vi "run.vi"() -> ()   [LabVIEW 2017]
uses:
  <vilib>/Analysis/Matrix/Datatypes/RealMatrix.ctl
  <vilib>/Simulation/Scripting/Companion Diagram/SimConfigNode/SimParams.ctl
  <vilib>/Simulation/Scripting/Companion Diagram/SimConfigNode/_simSolvers.ctl
  <vilib>/Simulation/Implementation/Shared/SIMSCR Execution Mode.ctl
  <vilib>/Simulation/Param Hierarchy/Typedefs/SIMPH Param Control Actions.ctl
  <vilib>/Simulation/Implementation/Shared/NILVSim_ParamChanged.vi
  <vilib>/Simulation/Implementation/Shared/NILVSIM_BeginStep.vi
  <vilib>/Simulation/SignalDisplay/Implementation/NILVSim Time Waveform.llb/SIM Time Waveform (vector).vi
  <vilib>/Simulation/SignalDisplay/Implementation/NILVSim Time Waveform.llb/SIM Time Waveform (scalar).vi
  <vilib>/Simulation/Implementation/Shared/SIM Is Init or Final Stage.vi
  <vilib>/Simulation/Implementation/Shared/NILVSim_Manager.vi
  <vilib>/Utility/error.llb/Clear Errors.vi
  <vilib>/Simulation/Implementation/Shared/NILVSim_FinalizeModel.vi
  <vilib>/picture/3D Picture Control/Object/Create Object (name).vi
  <vilib>/Analysis/7linalg.llb/Create Special Real Matrix.vi
  <vilib>/addons/Control Design/_Stochastic Systems/Stochastic Systems.llb/CD Construct Stochastic Model (Numeric).vi
  <vilib>/Simulation/Implementation/Shared/SIM Unbundle Sim Info.vi
  <vilib>/Simulation/Implementation/Shared/NILVSim_Initialize.vi
  SubVI/disturbance.vi
  <vilib>/addons/Control Design/_Stochastic Systems/Stochastic Systems.llb/CD Construct Noise Model.vi
  <vilib>/addons/Control Design/_Stochastic Systems/Stochastic Systems.llb/CD Construct Noise Model (Numeric).vi
  <vilib>/addons/Control Design/_State Feedback Control/State Feedback Control.llb/CD Linear Quadratic Regulator.vi
  <vilib>/addons/Control Design/_State Feedback Control/State Feedback Control.llb/State Feedback Control SubVis/cd_Linear Quadratic Regulator.vi
  <vilib>/addons/Control Design/_Implementation/CD State Feedback Controller.vi
  <vilib>/addons/Control Design/_Implementation/CD State Feedback Controller (Multiple Outputs).vi
  <vilib>/Simulation/Utility/Implementation/NILVSim Get Time and IsAcceptedStep.vi
  <vilib>/Simulation/DiscreteLinear/Implementation/NILVSim Discrete Stochastic State Space.llb/SIM Discrete Stochastic State Space External Indirect Distributor Sim.vi
  SubVI/lib/instrument.vi
  SubVI/3DMotion.vi
  <vilib>/Simulation/Estimation/Implementation/NILVSim Discrete Kalman Filter.llb/SIM Disc KF Pred and Corr with Pred Gain with Checking Indirect Distributor Sim.vi
  <vilib>/Simulation/DiscreteLinear/Implementation/NILVSim Discrete Stochastic State Space.llb/SIM Discrete Stochastic State Space External Indirect Collector Sim.vi
  <vilib>/Simulation/Estimation/Implementation/NILVSim Discrete Kalman Filter.llb/SIM Disc KF Pred and Corr with Pred Gain with Checking Indirect Collector Sim.vi
  <vilib>/Simulation/Implementation/Shared/SIMSH Read Queue.vi
  <vilib>/Simulation/Implementation/Shared/NILVSim_GetModelError.vi
  <vilib>/Simulation/Implementation/Shared/SIM Bundle Sim Info.vi
  <vilib>/Simulation/Scripting/Companion Diagram/SimConfigNode/SimDog.xnode
  <vilib>/Simulation/Implementation/XNodeFramework/SimXNode/SimX.xnode
  <vilib>/picture/3D Picture Control/NI_3D Picture Control.lvlib
  <vilib>/addons/Control Design/_State Feedback Control/NI_CD_State Feedback Control.lvlib
  <vilib>/addons/Control Design/_Stochastic Systems/NI_CD_Stochastic Systems.lvlib
  <vilib>/Analysis/NI_AALPro.lvlib
  <vilib>/addons/Control Design/_Utility/NI_CD_Model Viewer.lvlib
  <vilib>/addons/Control Design/_Implementation/NI_CD_Implementation.lvlib
  <vilib>/Simulation/Estimation/Implementation/NILVSim Discrete Kalman Filter.llb/SIM Disc KF Pred and Corr with Pred Gain with Checking Indirect Sim.vi
  <vilib>/Simulation/DiscreteLinear/Implementation/NILVSim Discrete Stochastic State Space.llb/NILVSim Discrete Stochastic State Space External Indirect Sim.vi
  <vilib>/Simulation/Implementation/Shared/NI_SIM_Implementation.lvlib
  <vilib>/Analysis/Matrix/NI_Matrix.lvlib
panel:
  in  "Optimal States (x1, x2, x3, x4, x5, x6)":dbl[](array[knob])=[1.0, 1.0, 1.0, 1.0, 1.0, 1.0] scale=0.01..100.0
  in  "Optimal Energy (u1, u2, u3)":dbl[](array[knob])=[1.0, 1.0, 1.0] scale=0.01..100.0
  out "State x(k+1)":dbl[](array[numeric])
  in  "Jz":dbl=0.0071
  in  "Jy":dbl=0.0038
  in  "Jx":dbl=0.0038
  in  "kr":dbl=0.00064
  in  "Pitch":dbl[](array[slide])=[0.0] scale=-30.0..60.0
  in  "Roll":dbl[](array[slide])=[0.0] scale=-89.0..89.0
  in  "Yaw S.P.":dbl[](array[slide])=[0.0] scale=-179.0..179.0
  in  "Orientation-Rate":dbl[](array[slide])=[0.0, 0.0, 0.0] scale=0.0..10.0
  out "Control Signals":waveform(dbl)[](graph)
  out "output cluster":T1 {"rotate"."pitch" scale=-30.0..60.0; "rotate"."roll" scale=-89.0..89.0; "rotate"."yaw" scale=-179.0..179.0}
  out "Yaw Error":waveform(dbl)[](graph)
  out "Pitch Error":waveform(dbl)(graph)={"t0"=timestamp(9343.2 s since 1904-01-01), "dt"=1.0, "Y"=[0.2633720690985406]}
  out "Roll Error":waveform(dbl)(graph)={"t0"=timestamp(9343.2 s since 1904-01-01), "dt"=1.0, "Y"=[0.2633720690985406]}
  out "Process Noise w(k)":dbl[](array[numeric])
  in  "Tab Control":enum32{"Model", "LQG"}(tab)
  out "Equation":picture
  out "Controller Action":dbl[](array[numeric]) format="%#.2g"
  out "Rv":T2
  in  "Convariance V":dbl(slide)=0.96 scale=0.0..1.0
  in  "Convariance W":dbl(slide)=0.96 scale=0.0..1.0
  out "Qw":T2
  in  "E{v}":dbl[](array[knob])=[0.96, 0.96, 0.96] scale=0.0..1.0
  in  "E{w}":dbl[](array[knob])=[0.96, 0.96, 0.96] scale=0.0..1.0
  in  "Initialize":bool
  out "Output y(t)":dbl[](array[numeric])
  out "Estimate xhat(k|k)":dbl[](array[numeric])
  out "Action u(k)":dbl[](array[numeric]) format="%#.2g"
  in  "Boolean 3":bool
  out "D(k)":dbl[](array[numeric])
  out "Setpoints_":dbl[](array[numeric])
  out "Yaw S.P. 2":dbl
  out "Waveform Yaw":waveform(dbl)[](graph)
  out "Waveform Pitch":waveform(dbl)[](graph)
  out "Pitch S.P.":dbl
  out "Roll S.P.":dbl
  out "Roll P.V.":dbl
  out "Waveform Roll":waveform(dbl)[](graph)
  in  "Switch\nController":bool
  out "pict out":picture
  out "Yaw P.V.":dbl
  out "Pitch P.V.":dbl
  out "3D Picture Control":refnum<vi>(3d-picture)
  # "References- Setpoints: Orientations, Angular Rates"
  # "N-Roll"
  # "N-Pitch"
  # "N-Yaw"
  # "Roll\nPitch\nYaw"
  # "Setpoints"
  # "u2\nu3 \nu4"
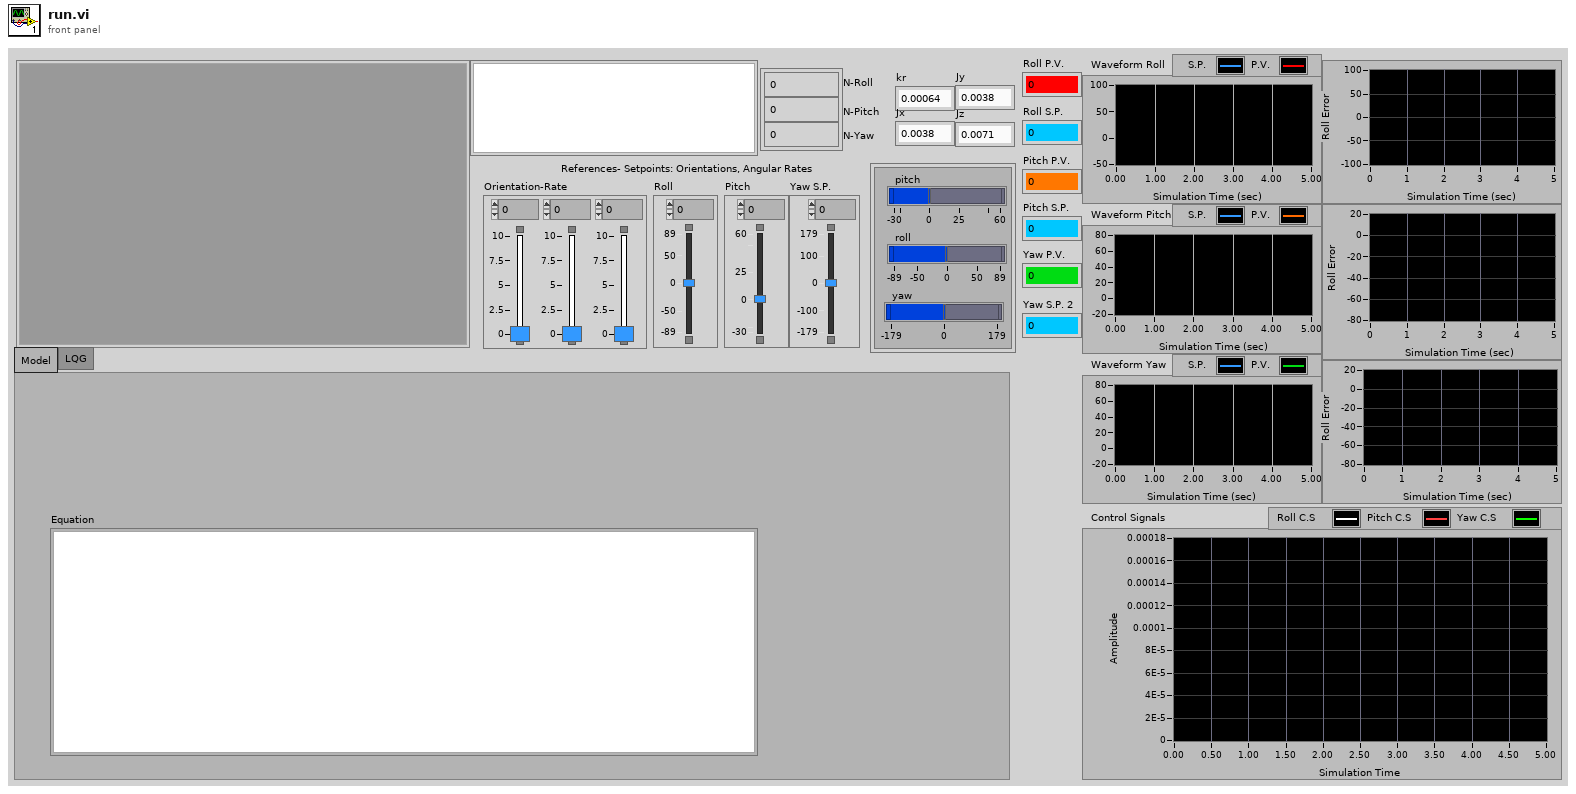
[diagram p1: front panel]
types:
  T1 = cluster{"control stick":cluster{"roll":i32, "pitch":i32}, "rotate":cluster{"pitch":dbl, "roll":dbl, "yaw":dbl}, "pos":cluster{"x":dbl, "y":dbl, "z":i32}}
  T2 = typedef "NI_Matrix.lvlib/RealMatrix.ctl" = dbl[][]
  T3 = typedef "NI_CD_Stochastic Systems.lvlib/cd_Stochastic State-Space Model.ctl" = cluster{"Sampling Time (s)":dbl, "G":dbl[][], "B":dbl[][], "A":dbl[][], "C":dbl[][], "D":dbl[][], "H":dbl[][]}
  T4 = typedef "NI_LinSys_Model Typedefs.lvlib/CD State Space Model (MIMO).ctl" = cluster{"properties":T5, "A":dbl[][], "B":dbl[][], "C":dbl[][], "D":dbl[][], "StateNames":string[], "Transport Delay":dbl[][]}
  T5 = typedef "NI_LinSys_Model Typedefs.lvlib/CD General Elements.ctl" = cluster{"Model name":string, "Input names":string[], "Output names":string[], "Input Delays":dbl[], "Output Delays":dbl[], "Sampling Time":dbl, "Notes":string}
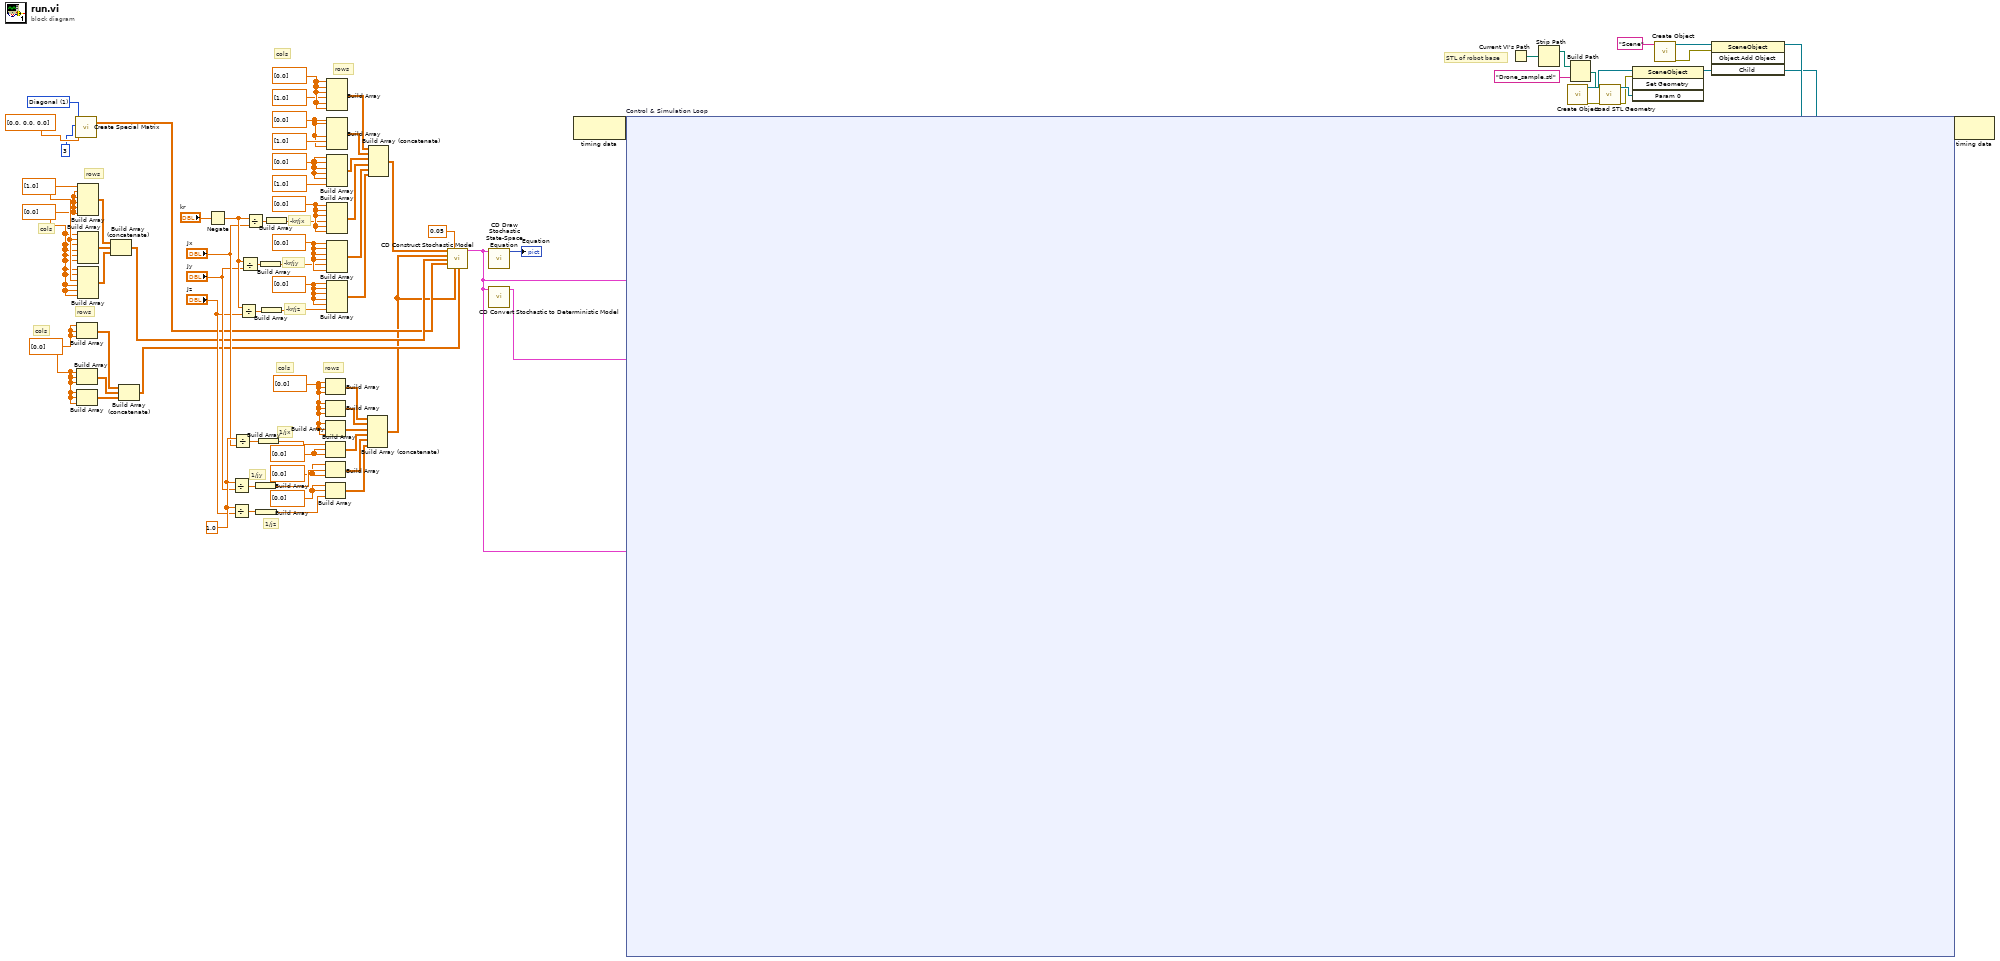
[diagram p0: block diagram]
diagram:
  w14 = dbl[] [0.0] ("element")
  w19 = dbl[] [1.0] ("element")
  w18 = dbl[] [0.0] ("element")
  w26 = 1 items=["Identity", "Diagonal", "Toepliz", "Vandermonde", "Companion", "Hankel", "Hadamard", "Wilkinson", "Hilbert", "Inverse Hilbert", "Rosser", "Pascal"] ("matrix type")
  w30 = 1.0 ("x")
  w34 = dbl[] [0.0] ("element")
  w35 = dbl[] [0.0] ("element")
  w36 = dbl[] [0.0] ("element")
  w20 = dbl[] [0.0] ("element")
  w59 = dbl[] [0.0] ("element")
  w58 = dbl[] [0.0] ("element")
  w57 = dbl[] [0.0] ("element")
  w63 = dbl[] [0.0] ("element")
  w65 = dbl[] [0.0] ("element")
  w68 = dbl[] [0.0] ("element")
  # "rows"
  # "cols"
  # "rows"
  # "cols"
  # "1/jz"
  # "1/jy"
  # "1/jx"
  # "rows"
  # "cols"
  # "-kr/jz"
  # "-kr/jy"
  # "-kr/jx"
  # "rows"
  # "cols"
  # "STL of robot base"
  n1 = call-poly <vilib>:"Create Special Matrix.vi"("matrix type"=w26, "matrix size"=3, "Input Vector1"=dbl[] [0.0, 0.0, 0.0]) -> ("Special Matrix"=w11:T2)  [unwired: 2 in, 1 out]
  n2 = Build Array(w14, w14, w14) -> (w17:T2)
  n3 = Build Array(w14, w14, w14) -> (w16:T2)
  n4 = Build Array(w14, w14, w14) -> (w15:T2)
  n5 = Build Array(w19, w18, w18, w18, w18, w18) -> (w21:T2)
  n6 = Build Array(w18, w19, w18, w18, w18, w18) -> (w22:T2)
  n7 = Build Array(w18, w18, w19, w18, w18, w18) -> (w23:T2)
  n8 = Build Array (concatenate)(w21, w22, w23) -> (w12:T2)
  n9 = Build Array (concatenate)(w17, w16, w15) -> (w5:T2)
  n10 = Negate(x="kr") -> (-x=w52:dbl)
  n11 = Divide(x=w30, y="Jy") -> (x/y=w43:dbl)
  n12 = Divide(x=w30, y="Jz") -> (x/y=w42:dbl)
  n13 = Divide(x=w30, y="Jx") -> (x/y=w40:dbl)
  n14 = Divide(x=w52, y="Jz") -> (x/y=w49:dbl)
  n15 = Divide(x=w52, y="Jy") -> (x/y=w48:dbl)
  n16 = Divide(x=w52, y="Jx") -> (x/y=w51:dbl)
  n17 = Build Array(w43) -> (w44:dbl[])
  n18 = Build Array(w42) -> (w45:dbl[])
  n19 = Build Array(w40) -> (w41:dbl[])
  n20 = Build Array(w48) -> (w47:dbl[])
  n21 = Build Array(w49) -> (w46:dbl[])
  n22 = Build Array(w51) -> (w50:dbl[])
  n23 = Build Array(w20, w20, w20) -> (w33:T2)
  n24 = Build Array(w20, w20, w20) -> (w32:T2)
  n25 = Build Array(w20, w20, w20) -> (w31:T2)
  n26 = Build Array(w41, w36, w36) -> (w37:T2)
  n27 = Build Array(w35, w44, w35) -> (w38:T2)
  n28 = Build Array(w34, w34, w45) -> (w39:T2)
  n29 = Build Array(w68, w68, w68, dbl[] [1.0] ("element"), w68, w68) -> (w60:T2)
  n30 = Build Array(w65, w65, w65, w65, dbl[] [1.0] ("element"), w65) -> (w61:T2)
  n31 = Build Array(w63, w63, w63, w63, w63, dbl[] [1.0] ("element")) -> (w62:T2)
  n32 = Build Array(w57, w57, w57, w50, w57, w57) -> (w56:T2)
  n33 = Build Array(w58, w58, w58, w58, w47, w58) -> (w55:T2)
  n34 = Build Array(w59, w59, w59, w59, w59, w46) -> (w54:T2)
  n35 = Build Array (concatenate)(w33, w32, w31, w37, w38, w39) -> (w4:T2)
  n36 = Build Array (concatenate)(w60, w61, w62, w56, w55, w54) -> (w13:T2)
  n37 = call-poly <vilib>:"CD Construct Stochastic Model.vi"("A"=w13, "Sampling Time (s)"=0.05, "B"=w4, "C"=w12, "D"=w11, "G"=w4, "H"=w5) -> ("Stochastic State-Space Model"=w2:T3)  [unwired: 7 in, 1 out]
  n38 = call <vilib>:"CD Draw Stochastic State-Space Equation.vi"("Stochastic State-Space Model"=w2) -> ("Equation"=→"Equation":picture)  [unwired: 8 in, 2 out]
  n39 = call <vilib>:"CD Convert Stochastic to Deterministic Model.vi"("Stochastic State-Space Model"=w2) -> ("Deterministic State-Space Model"=w1:T4)  [unwired: 13 in, 1 out]
  n40 = node-c288() -> (w7:variant)  [unwired: 1 in]
  n41 = Current VI's Path() -> (path=w71:path)
  n42 = Strip Path(path=w71) -> (stripped path=w70:path)  [unwired: 1 out]
  n43 = call-poly <vilib>:"Create Object.vi"() -> ("error out"=w75:errorcluster, "Scene:New Object"=w76:refnum<vi>)  [unwired: 10 in]
  n44 = Build Path(base path=w70, name or relative path="Drone_sample.stl") -> (appended path=w77:path)
  n45 = call <vilib>:"Load STL Geometry.vi"("error in (no error)"=w75, "Model File"=w77) -> ("error out"=w8:errorcluster, "New Mesh Refnum"=w9:refnum<vi>)  [unwired: 8 in]
  n46 = invoke class="SceneObject" method="Set Geometry"(reference=w76, error in=w8, "Param 0"=w9) -> (reference out=w74:refnum<vi>)  [unwired: 1 in, 3 out]
  n47 = call-poly <vilib>:"Create Object.vi"("Name"="Scene") -> ("error out"=w80:errorcluster, "Scene:New Object"=w79:refnum<vi>)  [unwired: 9 in]
  n48 = invoke class="SceneObject" method="Object.Add Object"(reference=w79, error in=w80, "Child"=w74) -> (reference out=w72:refnum<vi>, "Child"=w69:refnum<vi>)  [unwired: 1 in, 2 out]
  n49 = node-c254 "Control & Simulation Loop"(w7, w72, w69, w2, w1, w2) -> (w6:variant)
  n50 = node-c288(w6) -> ()  [unwired: 1 out]
